vi "ReadGFGandWriteToINI.vi"(8 "error in (no error)":errorcluster, 11 "Path":path) -> (0 "error out":errorcluster)   [LabVIEW 2012]
doc: "This VI reads an INI file and stores all keys in a Generalized Functional Global Variable (GFG). It then monitors updates to the GFG and writes keys back into INI file before closing. Note that the INI file only supports data type DBL or STRING. The GFG can handle any arbitrary data type, but values that are not DBL or STRING are discarded when closing and not written to INI file."
uses:
  GFG/GFGpathGet.vi
  <vilib>/Utility/config.llb/Write Key (Double).vi
  <vilib>/Utility/config.llb/Write Key (String).vi
  <vilib>/Utility/config.llb/Write Key (Boolean).vi
  <vilib>/Utility/config.llb/NI_LVConfig.lvlib
  GFG/GFG library.lvlib
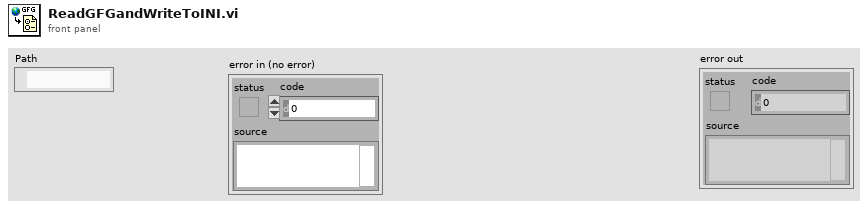
[diagram p1: front panel]
types:
  T1 = typedef "NI_LVConfig.lvlib/Config Data RefNum.ctl" = refnum<k1>
  T2 = typedef "VariantType.lvlib/Type.ctl" = enum8{"Invalid Type", "Void", "I8", "I16", "I32", "I64", "U8", "U16", "U32", "U64", "Single Float", "Double Float", "Extended Float", "Single Complex", "Double Complex", "Extended Complex", "Enum U8", "Enum U16", "Enum U32", "Enum U64", "Single Float With Unit", "Double Float With Unit", "Extended Float With Unit", "Single Complex with Unit", "Double Complex with Unit", "Extended Complex with Unit", "Boolean", "String", "Path", "Picture", "Tag", "Array", "Cluster", "Variant", "LV Variant", "Waveform", "Timestamp", "Digital Waveform", "Digital Data", "ExpressData", "Refnum", "External Data", "VI", "Poly VI", "LabVIEW Class Instance", "Fixed Point"}
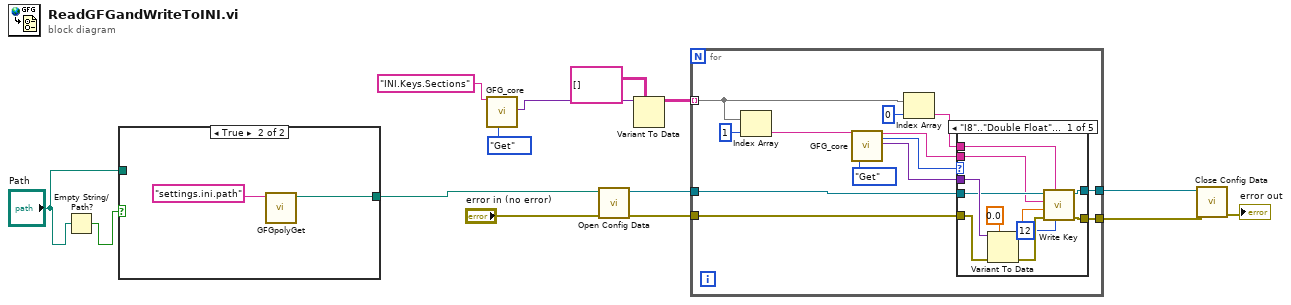
[diagram p0: block diagram]
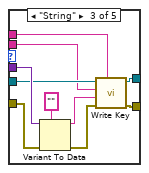
[diagram p4: hidden frame]
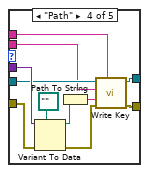
[diagram p5: hidden frame]
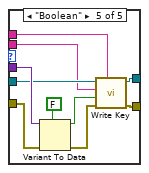
[diagram p6: hidden frame]
diagram:
  n1 = Empty String/Path?(string/path="Path") -> (empty?=w1:bool)
  n2 = case shown="True" w1 {
    tunnel: [w15 w16] -> w3
    tunnel: "Path" -> [w15 _]
    frame False {
    }
    frame True {
      n3 = call-poly "GFGpolyGet.vi"("Variable Name in"="settings.ini.path") -> ("Path"=w16:path)  [unwired: 9 in, 1 out]
    }
  }
  n4 = call "GFG_core.vi"("Variable Name in"="INI.Keys.Sections", "Action"=enum16{"Init", "Set", "Get"}."Get") -> ("Variant Out"=w11:variant)  [unwired: 11 in, 6 out]
  n5 = call <vilib>:"Open Config Data.vi"("error in (no error)"="error in (no error)", "configuration file path"=w3) -> ("error out"=w7:errorcluster, "refnum"=w8:T1)  [unwired: 7 in, 1 out]
  n6 = Variant To Data(type=string[][] [], Variant=w11) -> (data=w9:string[][])  [unwired: 1 in, 1 out]
  n7 = for {
    tunnel: w9 -> [w28] mode=indexing
    tunnel: [w22] -> w4
    tunnel: w8 -> [w21]
    tunnel: w7 -> [w23]
    tunnel: [w20] -> w5
    n8 = Index Array(array=w28, index=1) -> (element=w26:string)
    n9 = call "GFG_core.vi"("Variable Name in"=w26, "Action"=enum16{"Init", "Set", "Get"}."Get") -> ("Variable Name Out"=w19:string, "Data Type Out"=w25:T2, "Variant Out"=w24:variant)  [unwired: 11 in, 4 out]
    n10 = Index Array(array=w28, index=0) -> (element=w18:string)
    n11 = case shown="\"I8\"..\"Double Float\", \"Enum U8\"..\"Enum U64\"" w25 {
      tunnel: w24 -> [w40 _ w53 w64 w74]
      tunnel: [w37 w43 w50 w62 w71] -> w22
      tunnel: w23 -> [w36 w43 w49 w61 w70]
      tunnel: w21 -> [w35 w42 w48 w60 w69]
      tunnel: [w34 w42 w47 w59 w68] -> w20
      tunnel: w19 -> [w33 _ w46 w58 w67]
      tunnel: w18 -> [w32 _ w45 w57 w66]
      frame "I8".."Double Float", "Enum U8".."Enum U64" {
        n12 = Variant To Data(error in=w36, type=0.0, Variant=w40) -> (data=w39:dbl, error out=w38:errorcluster)
        n13 = call-poly <vilib>:"Write Key.vi"("precision (6)"=i16 12, "section"=w32, "error in (no error)"=w38, "value"=w39, "key"=w33, "refnum"=w35) -> ("error out"=w37:errorcluster, "refnum out"=w34:T1)  [unwired: 3 in, 1 out]
      }
      frame Default {
      }
      frame "String" {
        n14 = Variant To Data(error in=w49, type="" ("Variable Name Out"), Variant=w53) -> (data=w52:string, error out=w51:errorcluster)
        n15 = call-poly <vilib>:"Write Key.vi"("section"=w45, "error in (no error)"=w51, "value"=w52, "key"=w46, "refnum"=w48) -> ("error out"=w50:errorcluster, "refnum out"=w47:T1)  [unwired: 4 in, 1 out]
      }
      frame "Path" {
        n16 = Variant To Data(error in=w61, type=path "" ("configuration file path 2"), Variant=w64) -> (data=w54:path, error out=w63:errorcluster)
        n17 = Path To String(path=w54) -> (string=w55:string)
        n18 = call-poly <vilib>:"Write Key.vi"("section"=w57, "error in (no error)"=w63, "value"=w55, "key"=w58, "refnum"=w60) -> ("error out"=w62:errorcluster, "refnum out"=w59:T1)  [unwired: 4 in, 1 out]
      }
      frame "Boolean" {
        n19 = Variant To Data(error in=w70, type=FALSE, Variant=w74) -> (data=w73:bool, error out=w72:errorcluster)
        n20 = call-poly <vilib>:"Write Key.vi"("section"=w66, "error in (no error)"=w72, "value"=w73, "key"=w67, "refnum"=w69) -> ("error out"=w71:errorcluster, "refnum out"=w68:T1)  [unwired: 4 in, 1 out]
      }
    }
  }
  n21 = call <vilib>:"Close Config Data.vi"("error in (no error)"=w4, "refnum"=w5) -> ("error out"=→"error out":errorcluster)  [unwired: 8 in, 1 out]
